vi "Nome_Arquivo.vi"(6 "formato":string, 8 "Numeric 3":dbl, 9 "Numeric 2":dbl, 10 "Numeric":dbl, 11 "Path":path) -> (2 "path":path, 3 "String":string)   [LabVIEW 2019]
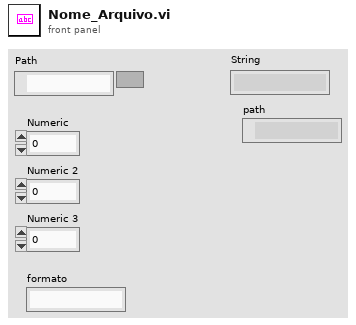
[diagram p1: front panel]
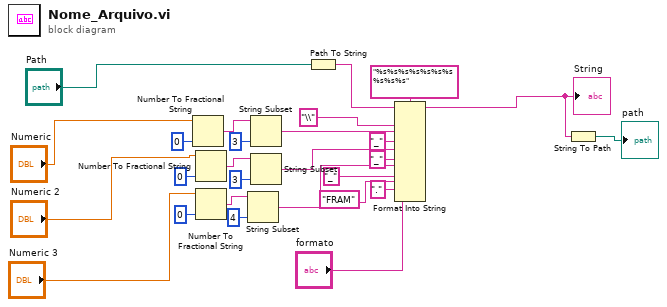
[diagram p0: block diagram]
diagram:
  n1 = Number To Fractional String(number="Numeric", precision (6)=i16 0) -> (F-format string=w16:string)  [unwired: 2 in]
  n2 = Number To Fractional String(number="Numeric 2", precision (6)=i16 0) -> (F-format string=w15:string)  [unwired: 2 in]
  n3 = Number To Fractional String(number="Numeric 3", precision (6)=i16 0) -> (F-format string=w14:string)  [unwired: 2 in]
  n4 = String Subset(string=w14, length (rest)=4 ("length (rest)")) -> (substring=w8:string)  [unwired: 1 in]
  n5 = String Subset(string=w16, length (rest)=3 ("length (rest)")) -> (substring=w10:string)  [unwired: 1 in]
  n6 = String Subset(string=w15, length (rest)=3 ("length (rest)")) -> (substring=w9:string)  [unwired: 1 in]
  n7 = Path To String(path="Path") -> (string=w27:string)
  n8 = Format Into String(format string="%s%s%s%s%s%s%s%s%s%s", initial string=w27, "\\" ("input 1"), w10, "_" ("input 3"), w9, "_" ("input 5"), w8, "_" ("input 7"), "FRAM" ("input 8"), "." ("input 9"), "formato") -> (resulting string=w2:string)  [unwired: 1 in, 1 out]
  "String" <- w2
  n9 = String To Path(string=w2) -> (path=→"path":path)
